vi "FTW-ActorExtended-Connection-Get.vi"(0 "FTW-ActorExtended In":refnum<class "FTW-ActorExtended.lvclass">, 5 "Connector Name":string, 11 "error in":errorcluster) -> (4 "FTW-ActorExtended Out":refnum<class "FTW-ActorExtended.lvclass">, 6 "FTW Actor Connector":refnum<class "FTW-ActorConnector.lvclass">, 15 "error out":errorcluster)   [LabVIEW 2015, in "FTW-ActorExtended.lvclass"]
uses:
  FTW-ActorExtended.lvclass
  Connector/FTW-ActorConnector.lvclass
  FTW-ActorExtended.lvclass/FTW-ActorExtended.ctl
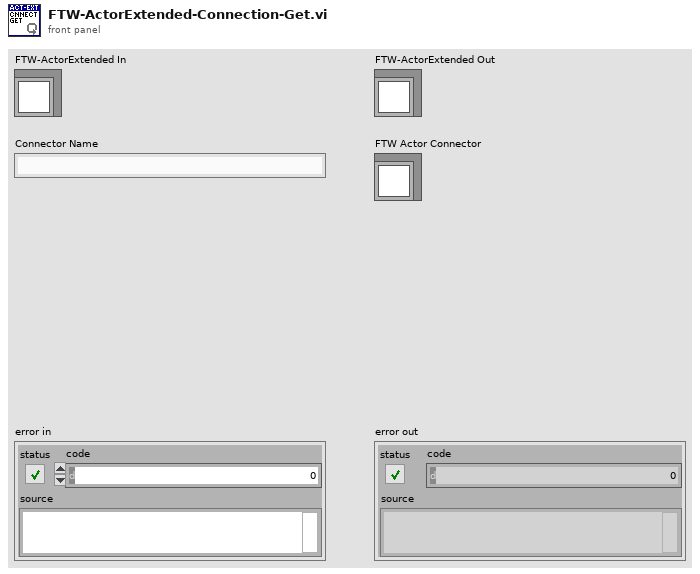
[diagram p1: front panel]
types:
  T1 = cluster{"Name":string, "URI":string, "Connector":refnum<class "FTW-ActorConnector.lvclass">, "Child":bool}[]
  T2 = cluster{"Name":string, "URI":string, "Connector":refnum<class "FTW-ActorConnector.lvclass">, "Child":bool}
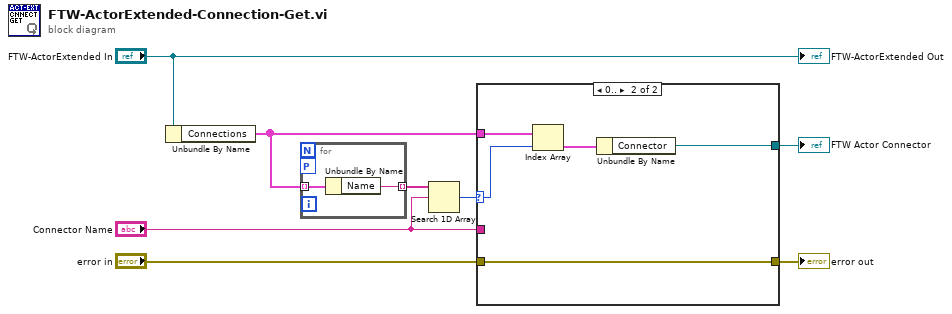
[diagram p0: block diagram]
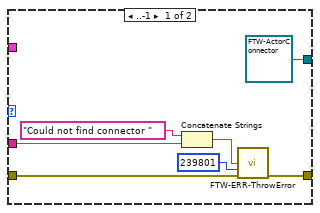
[diagram p2: hidden frame]
diagram:
  n1 = Unbundle By Name("FTW-ActorExtended In") -> ("Connections"=w6:T1)
  n2 = for {
    tunnel: w6 -> [w10] mode=indexing
    tunnel: [w9] -> w2 mode=indexing
    workers-P: _ -> [_]
    n3 = Unbundle By Name(w10) -> ("Name"=w9:string)
  }
  n4 = Search 1D Array(1D array=w2, element="Connector Name") -> (index of element=w7:i32)  [unwired: 1 in]
  n5 = case shown="0.." w7 {
    selector: w7 -> [_ w22]
    tunnel: w6 -> [_ w21]
    tunnel: [w16 w20] -> w5
    tunnel: "error in" -> [w17 w20]
    tunnel: "Connector Name" -> [w12 _]
    tunnel: [refnum<class "FTW-ActorConnector.lvclass"> refnum ("Connector") w18] -> w1
    frame ..-1 {
      n6 = Concatenate Strings("Could not find connector " ("Error Message"), w12) -> (w13:string)
      n7 = call "FTW-ERR-ThrowError.vi"("Error Message"=w13, "Error Code"=239801, "error in"=w17) -> ("error out"=w16:errorcluster)  [unwired: 12 in]
    }
    frame 0.. {
      n8 = Index Array(array=w21, index=w22) -> (element=w19:T2)
      n9 = Unbundle By Name(w19) -> ("Connector"=w18:refnum<class "FTW-ActorConnector.lvclass">)
    }
  }
  "error out" <- w5
  "FTW Actor Connector" <- w1
  "FTW-ActorExtended Out" <- "FTW-ActorExtended In"
